vi "TS Acq Stop.vi"(8 "error in":errorcluster, 11 "Test Stand in":refnum<class "Cryo Sep Test Stand.lvclass">) -> (0 "error out":errorcluster, 3 "Test Stand out":refnum<class "Cryo Sep Test Stand.lvclass">)   [LabVIEW 2019, in "Test Stands.lvlib" / "Cryo Sep Test Stand.lvclass"]
uses:
  Cryo Sep Test Stand.lvclass
  <vilib>/DAQmx/write.llb/DAQmx Write (Analog DBL 1Chan 1Samp).vi
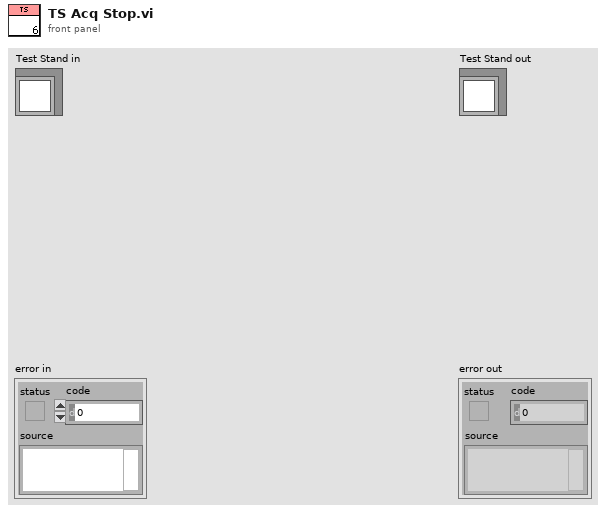
[diagram p1: front panel]
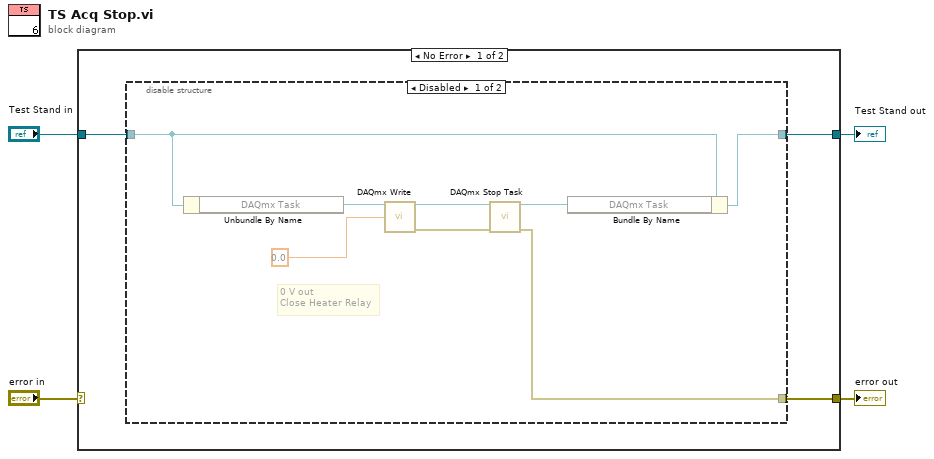
[diagram p0: block diagram]
diagram:
  n1 = case shown="No Error" "error in" {
    selector: "error in" -> [_ w18]
    tunnel: [w7 w18] -> w1
    tunnel: [w5 w17] -> w3
    tunnel: "Test Stand in" -> [w6 w17]
    frame No Error {
      n2 = disable-structure shown="Disabled" {
        disable-tunnel: [w11 _] -> w7
        disable-tunnel: w6 -> [w10 w16]
        disable-tunnel: [w8 w16] -> w5
        frame Disabled {
          # "0 V out\nClose Heater Relay"
          n3 = Unbundle By Name(w10) -> ("DAQmx Task"=w14:refnum<k21>)
          n4 = call-poly <vilib>:"DAQmx Write.vi"("task/channels in"=w14, "data"=0.0) -> ("task out"=w13:refnum<k21>, "error out"=w12:errorcluster)  [unwired: 11 in, 1 out]
          n5 = call <vilib>:"DAQmx Stop Task.vi"("task/channels in"=w13, "error in"=w12) -> ("task out"=w9:refnum<k21>, "error out"=w11:errorcluster)  [unwired: 12 in]
          n6 = Bundle By Name(cluster=w10, "DAQmx Task"=w9) -> (w8:refnum<class "Cryo Sep Test Stand.lvclass">)
        }
        frame Enabled {
        }
      }
    }
    frame Error {
    }
  }
  "error out" <- w1
  "Test Stand out" <- w3
